vi "Set or unset error -1210.vi"(6 "ID Control Refnum":refnum<vi>, 8 "error in":errorcluster, 9 "New Default Value":dbl, 10 "# of columns":i32, 11 "Item Ref In":T1 format="%.0x") -> (0 "error out":errorcluster, 3 "Item Ref Out":T1 format="%.0x")   [LabVIEW 2023, in "Vires VTD System Explorer.lvlib"]
uses:
  Vires VTD System Explorer.lvlib
  <vilib>/NI VeriStand/Custom Device API/Custom Device Item Ref.ctl
  <vilib>/NI VeriStand/Custom Device API/Custom Device API.lvlib
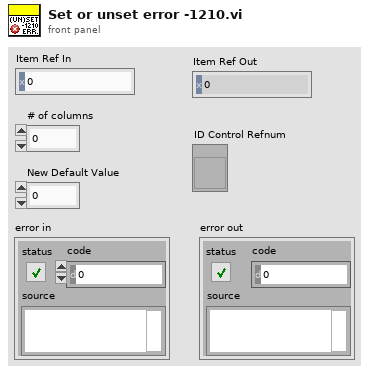
[diagram p1: front panel]
types:
  T1 = typedef "Custom Device API.lvlib/Custom Device Item Ref.ctl" = u64
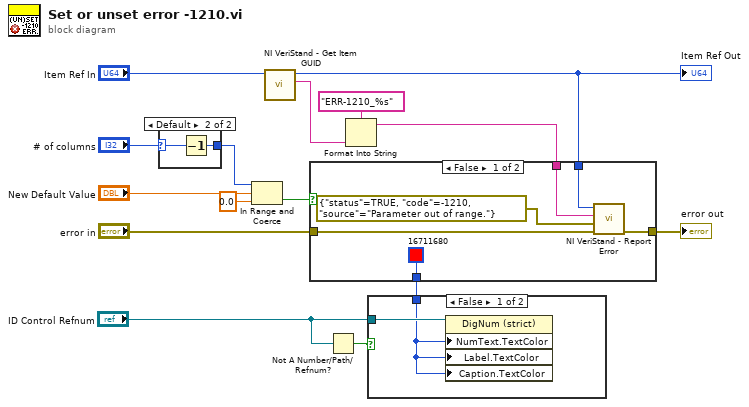
[diagram p0: block diagram]
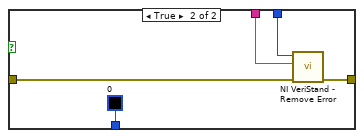
[diagram p3: hidden frame]
diagram:
  n1 = case shown="Default" "# of columns" {
    selector: "# of columns" -> [w16 w18]
    tunnel: [w16 w17] -> w11
    frame 0 {
    }
    frame Default {
      n2 = Decrement(x=w18) -> (x-1=w17:i32)
    }
  }
  n3 = In Range and Coerce(upper limit=w11, x="New Default Value", lower limit=0.0) -> (In Range?=w12:bool)  [unwired: 1 out]
  n4 = call <vilib>:"NI VeriStand - Get Item GUID.vi"("Item Ref in"="Item Ref In") -> ("GUID"=w6:string, "Item Ref out"=w7:T1)  [unwired: 8 in, 1 out]
  "Item Ref Out" <- w7
  n5 = Not A Number/Path/Refnum?(number/path/refnum="ID Control Refnum") -> (NaN/Path/Refnum?=w1:bool)
  n6 = Format Into String(format string="ERR-1210_%s", w6) -> (resulting string=w4:string)  [unwired: 2 in, 1 out]
  n7 = case shown="False" w12 {
    tunnel: "error in" -> [w24 w29]
    tunnel: w7 -> [w23 w27]
    tunnel: [w22 w28] -> w14
    tunnel: w4 -> [w21 w26]
    tunnel: [u32 16711680 u32 0] -> w3
    frame False {
      n8 = call <vilib>:"NI VeriStand - Report Error.vi"("error in (no error)"=w24, "New Error"=errorcluster {"status"=TRUE, "code"=-1210, "source"="Parameter out of range."}, "Error ID"=w21, "Node Ref in"=w23) -> ("error out"=w22:errorcluster)  [unwired: 6 in, 1 out]
    }
    frame True {
      n9 = call <vilib>:"NI VeriStand - Remove Error.vi"("error in (no error)"=w29, "Error ID"=w26, "Node Ref in"=w27) -> ("error out"=w28:errorcluster)  [unwired: 7 in, 1 out]
    }
  }
  "error out" <- w14
  n10 = case shown="False" w1 {
    tunnel: "ID Control Refnum" -> [w31 _]
    tunnel: w3 -> [w30 _]
    frame False {
      n11 = property class="DigNum (strict)"(reference=w31, "NumText.TextColor"=w30, "Label.TextColor"=w30, "Caption.TextColor"=w30) -> ()  [unwired: 1 in, 2 out]
    }
    frame True {
    }
  }
